vi "PT3_Open.vi"(8 "error in":errorcluster, 11 "File Path":path) -> (0 "error out":errorcluster, 1 "Num Records":i32, 2 "Header":T2, 3 "refnum out":refnum<file>, 4 "Stop After (ms)":i32, 5 "Stop Reason":enum16{"timeover", "manual", "overflow"}(ring), 7 "Image Header":T1)   [LabVIEW 2011]
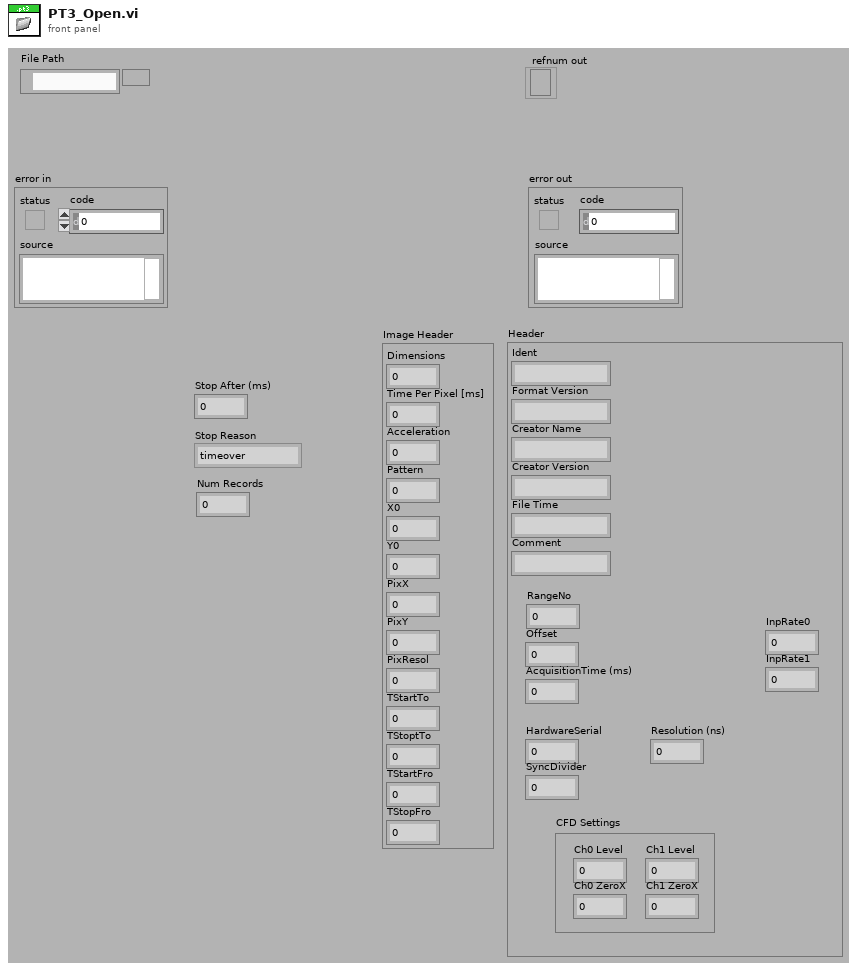
[diagram p1: front panel]
types:
  T1 = cluster{"Dimensions":i32, "Time Per Pixel [ms]":dbl, "Acceleration":i32, "Pattern":i32, "X0":sgl, "Y0":sgl, "PixX":i32, "PixY":i32, "PixResol":sgl, "TStartTo":sgl, "TStoptTo":sgl, "TStartFro":sgl, "TStopFro":sgl}
  T2 = cluster{"Ident":string, "Format Version":string, "Creator Name":string, "Creator Version":string, "File Time":string, "Comment":string, "RangeNo":i32, "Offset":i32, "AcquisitionTime (ms)":i32, "HardwareSerial":i32, "SyncDivider":i32, "Resolution (ns)":sgl, "CFD Settings":cluster{"Ch0 Level":i32, "Ch0 ZeroX":i32, "Ch1 Level":i32, "Ch1 ZeroX":i32}, "InpRate0":i32, "InpRate1":i32}
  T3 = enum16{"big-endian, network order", "native, host order", "little-endian"}
  T4 = enum16{"open", "replace", "create", "open or create", "replace or create", "replace or create with confirmation"}
  T5 = cluster{"Strings[0]":string, "Strings[1]":string, "Strings[2]":string, "Strings[3]":string, "Strings[4]":string, "Strings[5]":string}
  T6 = cluster{"[0]":i32, "[1]":i32, "[2]":i32, "[3]":i32, "[4]":i32, "[5]":i32}
  T7 = cluster{"[3]":i32, "[2]":i32, "[5]":i32, "[4]":i32}
  T8 = cluster{"[0]":i32, "[1]":i32, "[2]":i32, "[3]":i32, "[4]":i32, "[5]":i32, "[6]":i32, "[7]":i32, "[8]":i32}
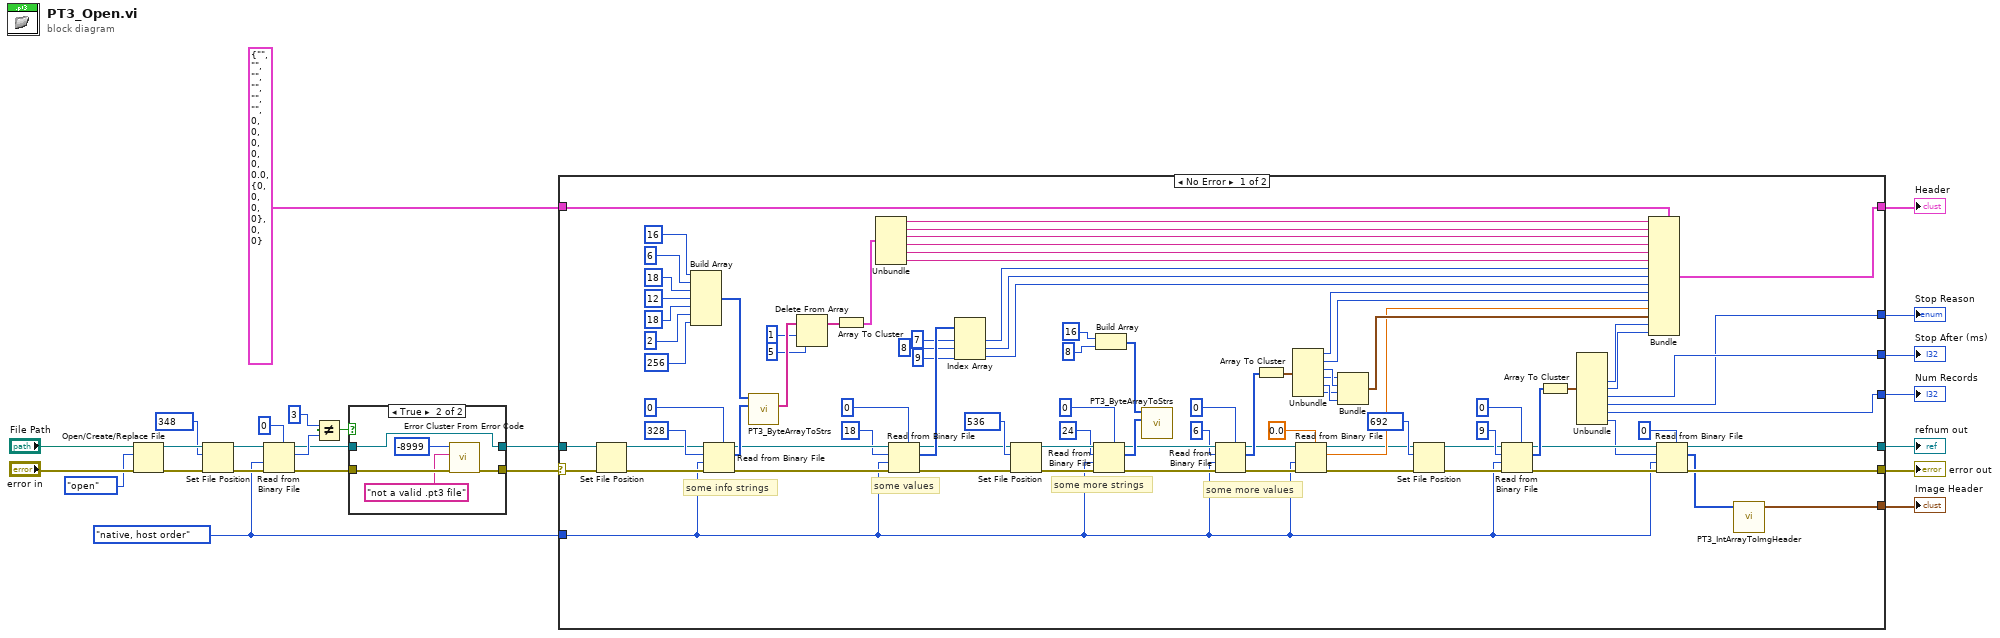
[diagram p0: block diagram]
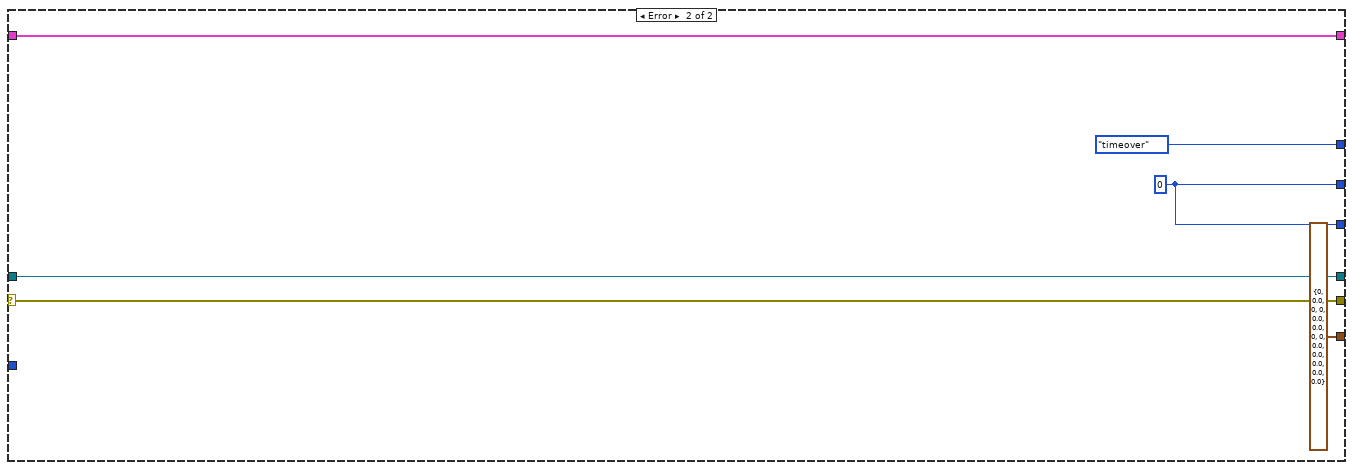
[diagram p3: hidden frame]
diagram:
  w11 = T3."native, host order" ("byte order (0:big-endian, network order)")
  n1 = Open/Create/Replace File(file path (use dialog)="File Path", error in="error in", operation (0:open)=T4."open") -> (refnum out=w14:refnum<file>, error out=w15:errorcluster)  [unwired: 4 out]
  n2 = Set File Position(offset (in bytes) (0)=i64 348, refnum=w14, error in=w15) -> (refnum out=w10:refnum<file>, error out=w12:errorcluster)  [unwired: 1 out]
  n3 = Read from Binary File(5:0, 8:w12, 9:w11, 11:w10) -> (0:w5:errorcluster, 2:w8:i32, 3:w2:refnum<file>)  [unwired: 3 out]
  n4 = Not Equal?(x=3, y=w8) -> (x != y?=w6:bool)
  n5 = case shown="True" w6 {
    tunnel: w5 -> [w27 w32]
    tunnel: [w27 w31] -> w4
    tunnel: [w26 w28] -> w3
    tunnel: w2 -> [w26 w28]
    frame False {
    }
    frame True {
      n6 = call <vilib>:"Error Cluster From Error Code.vi"("error in (no error)"=w32, "error message (\"\")"="not a valid .pt3 file" ("error message (\"\")"), "error code (0)"=-8999) -> ("error out"=w31:errorcluster)  [unwired: 1 in, 5 out]
    }
  }
  n7 = case shown="No Error" w4 {
    selector: w4 -> [w105 w128]
    tunnel: [w36 w128] -> w22
    tunnel: [w35 w127] -> w21
    tunnel: w3 -> [w103 w127]
    tunnel: w11 -> [w38 _]
    tunnel: [w94 w124] -> w20
    tunnel: [w42 enum16{"timeover", "manual", "overflow"}."timeover" ("Stop Reason")] -> w19
    tunnel: [w44 w125] -> w18
    tunnel: [w43 w125] -> w17
    tunnel: T2 {"Ident"="", "Format Version"="", "Creator Name"="", "Creator Version"="", "File Time"="", "Comment"="", "RangeNo"=0, "Offset"=0, "AcquisitionTime (ms)"=0, "HardwareSerial"=0, "SyncDivider"=0, "Resolution (ns)"=0.0, "CFD Settings"={"Ch0 Level"=0, "Ch0 ZeroX"=0, "Ch1 Level"=0, "Ch1 ZeroX"=0}, "InpRate0"=0, "InpRate1"=0} ("Header") -> [w95 w124]
    tunnel: [w33 T1 {"Dimensions"=0, "Time Per Pixel [ms]"=0.0, "Acceleration"=0, "Pattern"=0, "X0"=0.0, "Y0"=0.0, "PixX"=0, "PixY"=0, "PixResol"=0.0, "TStartTo"=0.0, "TStoptTo"=0.0, "TStartFro"=0.0, "TStopFro"=0.0} ("Image Header")] -> w1
    frame No Error {
      # "some more values"
      # "some more strings"
      # "some values"
      # "some info strings"
      n8 = Set File Position(refnum=w103, error in=w105) -> (refnum out=w102:refnum<file>, error out=w104:errorcluster)  [unwired: 2 out]
      n9 = Build Array(16 ("Length"), 6 ("Length"), 18 ("Length"), 12 ("Length"), 18 ("Length"), 2 ("Length"), 256 ("Length")) -> (w112:i32[])
      n10 = Read from Binary File(5:u8 0, 8:w104, 9:w38, 10:328 ("count (1)"), 11:w102) -> (0:w107:errorcluster, 2:w120:u8[], 3:w106:refnum<file>)  [unwired: 2 out]
      n11 = call "PT3_ByteArrayToStrs.vi"("Byte Array"=w120, "Lengths"=w112) -> ("Strings"=w111:string[])  [unwired: 9 out]
      n12 = Delete From Array(array=w111, length=1, index=5) -> (array with subset deleted=w108:string[])  [unwired: 1 out]
      n13 = Array To Cluster(array=w108) -> (cluster=w93:T5)
      n14 = Unbundle(w93) -> ("Strings[0]"=w92:string, "Strings[1]"=w91:string, "Strings[2]"=w90:string, "Strings[3]"=w89:string, "Strings[4]"=w88:string, "Strings[5]"=w87:string)
      n15 = Read from Binary File(5:0, 8:w107, 9:w38, 10:18 ("count (1)"), 11:w106) -> (0:w82:errorcluster, 2:w99:i32[], 3:w81:refnum<file>)  [unwired: 2 out]
      n16 = Index Array(array=w99, index #1=7 ("index"), index #2=8 ("index"), index #3=9 ("index")) -> (element #1=w86:i32, element #2=w85:i32, element #3=w84:i32)
      n17 = Set File Position(offset (in bytes) (0)=i64 536, refnum=w81, error in=w82) -> (refnum out=w79:refnum<file>, error out=w80:errorcluster)  [unwired: 1 out]
      n18 = Read from Binary File(5:u8 0, 8:w80, 9:w38, 10:24 ("count (1)"), 11:w79) -> (0:w72:errorcluster, 2:w76:u8[], 3:w71:refnum<file>)  [unwired: 2 out]
      n19 = Build Array(16 ("Length"), 8 ("Length")) -> (w73:i32[])
      n20 = call "PT3_ByteArrayToStrs.vi"("Byte Array"=w76, "Lengths"=w73) -> ()  [unwired: 10 out]
      n21 = Read from Binary File(5:0, 8:w72, 9:w38, 10:6 ("count (1)"), 11:w71) -> (0:w59:errorcluster, 2:w68:i32[], 3:w57:refnum<file>)  [unwired: 2 out]
      n22 = Array To Cluster(array=w68) -> (cluster=w67:T6)
      n23 = Unbundle(w67) -> ("[0]"=w66:i32, "[1]"=w65:i32, "[2]"=w64:i32, "[3]"=w63:i32, "[4]"=w62:i32, "[5]"=w61:i32)
      n24 = Read from Binary File(5:sgl 0.0 ("Resolution (ns)"), 8:w59, 9:w38, 11:w57) -> (0:w54:errorcluster, 2:w56:sgl, 3:w53:refnum<file>)  [unwired: 3 out]
      n25 = Bundle("[3]"=w63, "[2]"=w64, "[5]"=w61, "[4]"=w62) -> (w60:T7)  [unwired: 1 out]
      n26 = Set File Position(offset (in bytes) (0)=i64 692, refnum=w53, error in=w54) -> (refnum out=w49:refnum<file>, error out=w50:errorcluster)  [unwired: 1 out]
      n27 = Read from Binary File(5:0, 8:w50, 9:w38, 10:9 ("count (1)"), 11:w49) -> (0:w41:errorcluster, 2:w47:i32[], 3:w40:refnum<file>)  [unwired: 2 out]
      n28 = Array To Cluster(array=w47) -> (cluster=w48:T8)
      n29 = Unbundle(w48) -> ("[3]"=w46:i32, "[4]"=w45:i32, "[5]"=w44:i32, "[6]"=w42:i32, "[7]"=w43:i32, "[8]"=w37:i32)  [unwired: 3 out]
      n30 = Bundle(cluster=w95, "Ident"=w92, "Format Version"=w91, "Creator Name"=w90, "Creator Version"=w89, "File Time"=w88, "Comment"=w87, "RangeNo"=w86, "Offset"=w85, "AcquisitionTime (ms)"=w84, "HardwareSerial"=w66, "SyncDivider"=w65, "Resolution (ns)"=w56, "CFD Settings"=w60, "InpRate0"=w46, "InpRate1"=w45) -> (w94:T2)
      n31 = Read from Binary File(5:0, 8:w41, 9:w38, 10:w37, 11:w40) -> (0:w36:errorcluster, 2:w34:i32[], 3:w35:refnum<file>)  [unwired: 2 out]
      n32 = call "PT3_IntArrayToImgHeader.vi"("Array"=w34) -> ("Image Header"=w33:T1)  [unwired: 10 out]
    }
    frame Error {
      w125 = 0 ("Stop After (ms)")
    }
  }
  "refnum out" <- w21
  "error out" <- w22
  "Header" <- w20
  "Stop Reason" <- w19
  "Stop After (ms)" <- w18
  "Num Records" <- w17
  "Image Header" <- w1
